vi "Strip Trailing Zeros for Float String.vi"(11 "Float String":string) -> (3 "Float String with Same Value":string)   [LabVIEW 2017, in "API String Arguments Support.lvlib"]
uses:
  API String Arguments Support.lvlib
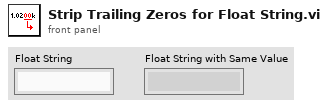
[diagram p1: front panel]
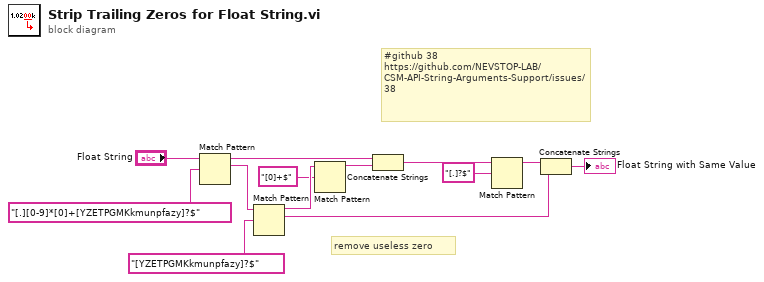
[diagram p0: block diagram]
diagram:
  # "#github 38\nhttps://github.com/NEVSTOP-LAB/CSM-API-String-Arguments-Support/issues/38"
  # "remove useless zero"
  n1 = Match Pattern(string="Float String", regular expression="[.][0-9]*[0]+[YZETPGMKkmunpfazy]?$") -> (before substring=w2:string, match substring=w5:string)  [unwired: 1 in, 2 out]
  n2 = Match Pattern(string=w5, regular expression="[YZETPGMKkmunpfazy]?$") -> (before substring=w8:string, match substring=w9:string)  [unwired: 1 in, 2 out]
  n3 = Match Pattern(string=w8, regular expression="[0]+$") -> (before substring=w6:string)  [unwired: 1 in, 3 out]
  n4 = Concatenate Strings(w2, w6) -> (w12:string)
  n5 = Match Pattern(string=w12, regular expression="[.]?$") -> (before substring=w13:string)  [unwired: 1 in, 3 out]
  n6 = Concatenate Strings(w13, w9) -> (→"Float String with Same Value":string)
